vi "DigSeqLogic_SR_FlipFlop.vi"(5 "Set":bool, 9 "Reset":bool, 13 "Initial Value":bool) -> (6 "Output":bool, 10 "Inverse Output":bool=TRUE)   [LabVIEW 2019, in "Trajectory_Library.lvlib"]
doc: "This VI implements a standard Set-Reset (SR) Flip Flop. A flip flop is sometimes called \"digital memory\" because when both inputs are off, it remembers the state of the last input.\n\nReset takes precedence over Set. The initial state is Reset. \n\nInputs:\n - Set -- Boolean, when TRUE indicates the flip-flop should be SET.\n - Reset -- Boolean, when TRUE indicates the flip-flop should be RESET. (Reset overrides set.)\n - InitialValue -- Value of the flip-flop during the first execution. TRUE = SET, FALSE = RESET. (Defaul: False)\n\nOutput:\n - Output -- Output state of the flip-flop\n - Inverse Output -- Inverse (NOT) output of the flip-flop."
uses:
  Trajectory_Library.lvlib
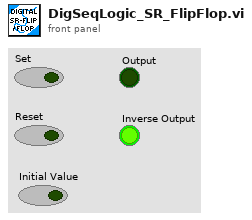
[diagram p1: front panel]
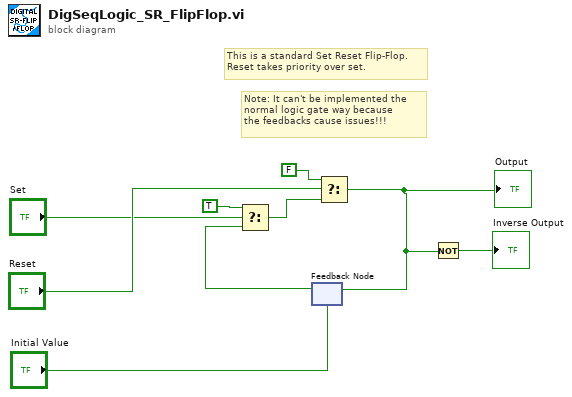
[diagram p0: block diagram]
diagram:
  # "Note: It can't be implemented the \nnormal logic gate way because\nthe feedbacks cause issues!!!"
  # "This is a standard Set Reset Flip-Flop.  \nReset takes priority over set."
  n1 = feedback #1("Initial Value") -> (w3:bool)
  n2 = Select(t=TRUE, s="Set", f=w3) -> (s? t:f=w5:bool)
  n3 = Select(t=FALSE, s="Reset", f=w5) -> (s? t:f=w1:bool)
  "Output" <- w1
  n4 = feedback-in #1(w1) -> ()
  n5 = Not(x=w1) -> (.not. x?=→"Inverse Output":bool)
